vi "逻辑门和七段共阴极数码管设计译码显示电路.vi"() -> ()   [LabVIEW 2018]
panel:
  in  "结束":bool
  out "dp":bool
  out "c":bool
  out "e":bool
  out "b":bool
  out "f":bool
  out "d":bool
  out "g":bool
  out "a":bool
  in  "S1":bool
  in  "S0":bool
  # "74HC00：与非门\n74HC04：非门"
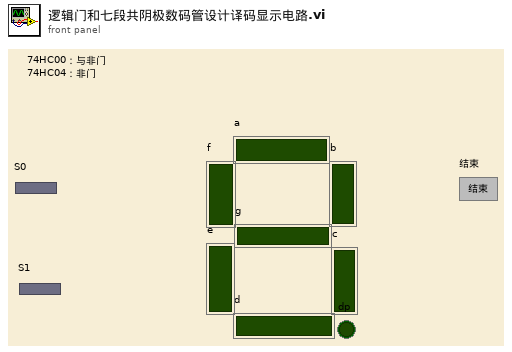
[diagram p1: front panel]
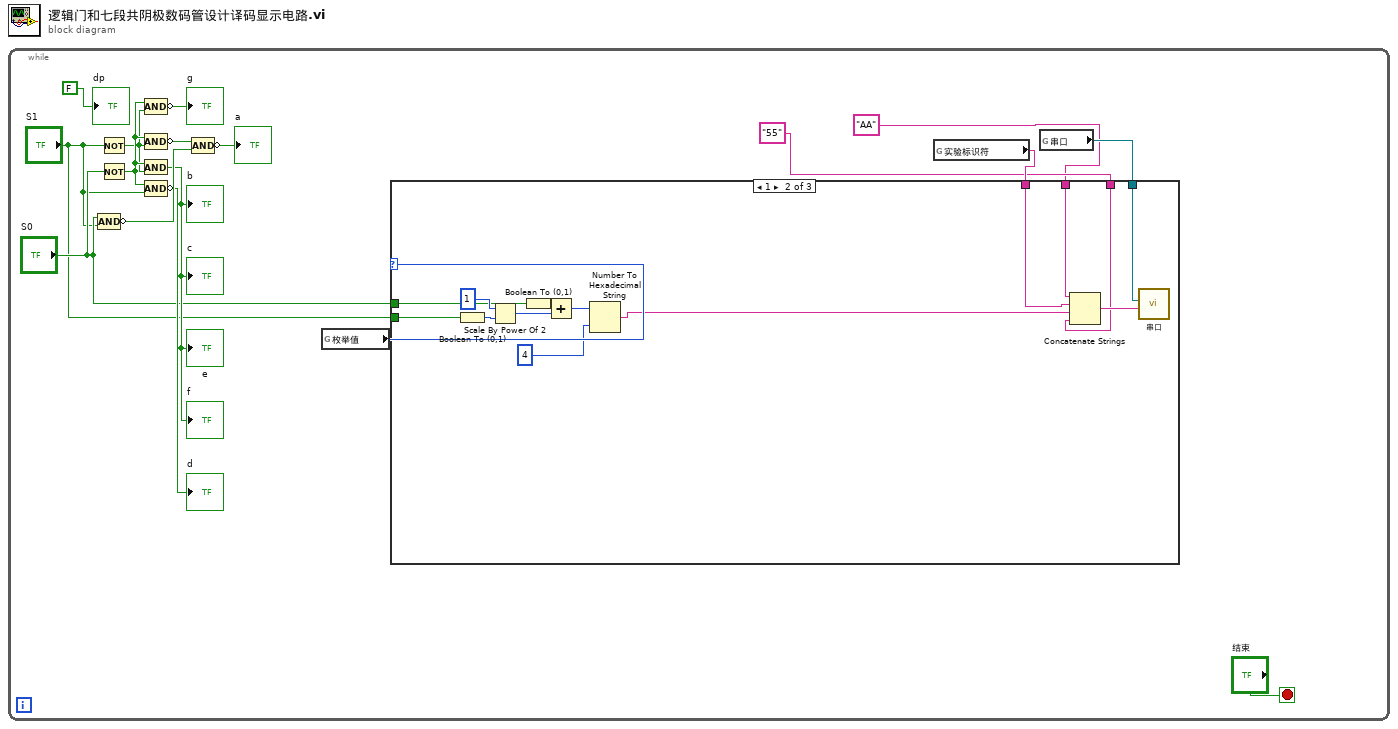
[diagram p0: block diagram]
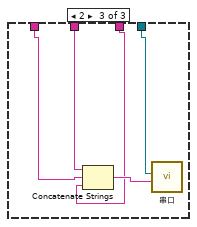
[diagram p3: hidden frame]
diagram:
  n1 = while {
    stop <- "结束" stop-if-true
    n2 = Compound Arithmetic op=AND ("复合运算")("S0", "S1") -> (invert w16:bool)
    n3 = Not(x="S1") -> (.not. x?=w11:bool)
    n4 = Not(x="S0") -> (.not. x?=w12:bool)
    n5 = And(x=w12, y=w11) -> (x .and. y?=→"f" →"b" →"e" →"c":bool)
    n6 = Compound Arithmetic op=AND ("复合运算")(w12, w11) -> (invert →"g":bool)
    n7 = Compound Arithmetic op=AND ("复合运算")(w12, w11) -> (invert w17:bool)
    n8 = Compound Arithmetic op=AND ("复合运算")(w12, "S1") -> (invert →"d":bool)
    n9 = Compound Arithmetic op=AND ("复合运算")(w17, w16) -> (invert →"a":bool)
    n10 = global read "全局变量.vi" "枚举值"() -> (w7:i8)
    n11 = global read "全局变量.vi" "实验标识符"() -> (w5:string)
    n12 = global read "全局变量.vi" "串口"() -> (w6:refnum<visa-resource-name>)
    n13 = case shown="1" w7 {
      tunnel: "S1" -> [_ w26 _]
      tunnel: "S0" -> [_ w25 _]
      tunnel: w6 -> [_ w24 w34]
      tunnel: w5 -> [_ w23 w35]
      tunnel: "55" -> [_ w22 w32]
      tunnel: "AA" -> [_ w21 w33]
      frame 0, Default {
      }
      frame 1 {
        n14 = Boolean To (0,1)(Boolean=w26) -> (0, 1=w28:i16)
        n15 = Scale By Power Of 2(n=1, x=w28) -> (x*2^n=w29:i16)
        n16 = Boolean To (0,1)(Boolean=w25) -> (0, 1=w30:i16)
        n17 = Add(x=w30, y=w29) -> (x+y=w20:i16)
        n18 = Number To Hexadecimal String(1:4, 2:w20) -> (0:w18:string)
        n19 = Concatenate Strings(w21, w23, w18, w22) -> (w31:string)
        n20 = call "串口.vi"("字符串"=w31, "VISA resource name"=w24) -> ()  [unwired: 10 in]
      }
      frame 2 {
        n21 = Concatenate Strings(w33, w35, w32) -> (w36:string)
        n22 = call "串口.vi"("字符串"=w36, "VISA resource name"=w34) -> ()  [unwired: 10 in]
      }
    }
    "dp" <- FALSE
  }
